vi "Version_2.0_Single_Column_Code.vi"() -> ()   [LabVIEW 2020] (continued)
                              frame #2 {
                                n5157 = local read "VISA Refnum in\nfor Pump"() -> (w5540:refnum<visa-resource-name>)
                                n5158 = call "PortChanger (SubVI).vi"("Port Number"="1", "VISA Refnum in"=w5540) -> ()  [unwired: 10 in]
                              }
                              frame #3 {
                                n5159 = local read "Stopper that ends \nthe main loops"() -> (w5541:bool)
                                n5160 = local read "VISA Refnum in\nfor Pump"() -> (w5542:refnum<visa-resource-name>)
                                n5161 = case shown="True" w5541 {
                                frame False {
                                }
                                frame True {
                                n5162 = local read "VISA Refnum in\nfor Pump"() -> (w5543:refnum<visa-resource-name>)
                                n5163 = call "HardStopCurrentProcess (SubVI).vi"("VISA Refnum in"=w5543) -> ()  [unwired: 11 in]
                                }
                                }
                                n5164 = call "ProcessCompletionWaiter (SubVI).vi"("VISA Refnum in"=w5542) -> ()  [unwired: 11 in]
                              }
                              frame #4 {
                                n5165 = local read "VISA Refnum in\nfor Pump"() -> (w5548:refnum<visa-resource-name>)
                                n5166 = local read "Volume of Syringe"() -> (w5545:dbl)
                                n5167 = call "GoToAbsolutePosition(SubVI).vi"("Absolute Volume Position in Syringe (in ul)"=0.0, "Volume of Syringe"=w5545, "Resolution of Pumping"=T2."Standard Pumping", "Flow Rate (ul/min)"=150.0, "VISA Refnum in"=w5548) -> ()  [unwired: 6 in, 1 out]
                              }
                              frame #5 {
                                n5168 = local read "Stopper that ends \nthe main loops"() -> (w5549:bool)
                                n5169 = local read "VISA Refnum in\nfor Pump"() -> (w5550:refnum<visa-resource-name>)
                                n5170 = case shown="True" w5549 {
                                frame False {
                                }
                                frame True {
                                n5171 = local read "VISA Refnum in\nfor Pump"() -> (w5551:refnum<visa-resource-name>)
                                n5172 = call "HardStopCurrentProcess (SubVI).vi"("VISA Refnum in"=w5551) -> ()  [unwired: 11 in]
                                }
                                }
                                n5173 = call "ProcessCompletionWaiter (SubVI).vi"("VISA Refnum in"=w5550) -> ()  [unwired: 11 in]
                              }
                            }
                          }
                          frame #3 {
                            n5174 = local read "VISA Refnum in\nfor Pump"() -> (w5553:refnum<visa-resource-name>)
                            n5175 = local read "Port for \nB-Elution"() -> (w5552:string)
                            n5176 = call "PortChanger (SubVI).vi"("Port Number"=w5552, "VISA Refnum in"=w5553) -> ()  [unwired: 10 in]
                          }
                          frame #4 {
                            n5177 = local read "VISA Refnum in\nfor Pump"() -> (w5554:refnum<visa-resource-name>)
                            n5178 = call "ProcessCompletionWaiter (SubVI).vi"("VISA Refnum in"=w5554) -> ()  [unwired: 11 in]
                          }
                          frame #5 {
                            n5179 = local read "Buffer-B PickUp \nFlow Rate (ul/min)"() -> (w5557:dbl)
                            n5180 = local read "Buffer-B Pumping\nResolution"() -> (w5556:T2)
                            n5181 = local read "VISA Refnum in\nfor Pump"() -> (w5559:refnum<visa-resource-name>)
                            n5182 = local read "Buffer-B Volume \nto be  Pumped"() -> (w5555:dbl)
                            n5183 = local read "Volume of Syringe"() -> (w5558:dbl)
                            n5184 = call "RPickUp(SubVI).vi"("Volume to be picked up"=w5555, "Volume of Syringe"=w5558, "Resolution of PickUP"=w5556, "PickUp Flow Rate (ul/min)"=w5557, "VISA Refnum in"=w5559) -> ()  [unwired: 6 in, 1 out]
                          }
                          frame #6 {
                            n5185 = local read "Stopper that ends \nthe main loops"() -> (w5560:bool)
                            n5186 = local read "VISA Refnum in\nfor Pump"() -> (w5561:refnum<visa-resource-name>)
                            n5187 = case shown="True" w5560 {
                              frame False {
                              }
                              frame True {
                                n5188 = local read "VISA Refnum in\nfor Pump"() -> (w5562:refnum<visa-resource-name>)
                                n5189 = call "HardStopCurrentProcess (SubVI).vi"("VISA Refnum in"=w5562) -> ()  [unwired: 11 in]
                              }
                            }
                            n5190 = call "ProcessCompletionWaiter (SubVI).vi"("VISA Refnum in"=w5561) -> ()  [unwired: 11 in]
                          }
                          frame #7 {
                            # "Reads the initial Plunger Position for computing the volume dispensed"
                            n5191 = local read "VISA Refnum in\nfor Pump"() -> (w5564:refnum<visa-resource-name>)
                            n5192 = call "AbsolutePlungerPosition (SubVI).vi"("VISA Refnum in"=w5564) -> ("Plunger Position"=w5563:i32)  [unwired: 10 in]
                            n5193 = local write "Initial Plunger Position"(w5563) -> ()
                          }
                          frame #8 {
                            # "Switch to Port-8"
                            # "Port-8 of the pump is conncted to elution port of column-1 of chip"
                            n5194 = local read "VISA Refnum in\nfor Pump"() -> (w5566:refnum<visa-resource-name>)
                            n5195 = call "PortChanger (SubVI).vi"("Port Number"="8", "VISA Refnum in"=w5566) -> ()  [unwired: 10 in]
                          }
                          frame #9 {
                            n5196 = local read "Stopper that ends \nthe main loops"() -> (w5567:bool)
                            n5197 = local read "VISA Refnum in\nfor Pump"() -> (w5568:refnum<visa-resource-name>)
                            n5198 = call "ProcessCompletionWaiter (SubVI).vi"("VISA Refnum in"=w5568) -> ()  [unwired: 11 in]
                            n5199 = case shown="True" w5567 {
                              frame False {
                              }
                              frame True {
                                n5200 = local read "VISA Refnum in\nfor Pump"() -> (w5569:refnum<visa-resource-name>)
                                n5201 = call "HardStopCurrentProcess (SubVI).vi"("VISA Refnum in"=w5569) -> ()  [unwired: 11 in]
                              }
                            }
                          }
                          frame #10 {
                            # "Discard first few microlitres of elution buffer"
                            # "Keeps the AMF valve after column-1 open and valve after column-2 closed"
                            n5202 = local write "Valve V1 Open"(FALSE ("Valve V1 Open")) -> ()
                            n5203 = local write "Valve V2 Open"(FALSE ("Valve V2 Open")) -> ()
                            n5204 = local write "Valve V3 Open"(FALSE ("Valve V3 Open")) -> ()
                            n5205 = local write "Valve V4 Open"(FALSE ("Valve V4 Open")) -> ()
                            n5206 = local write "External Valve \nOpen"(FALSE ("External Valve \nOpen")) -> ()
                            n5207 = local write "Valve V8 Open"(TRUE ("Valve V8 Open")) -> ()
                            n5208 = local write "Valve V6 Open"(FALSE ("Valve V6 Open")) -> ()
                            n5209 = local write "Valve V5 Open"(FALSE ("Valve V5 Open")) -> ()
                            n5210 = local write "Valve V7 Open"(FALSE ("Valve V7 Open")) -> ()
                          }
                          frame #11 {
                            n5211 = local read "Buffer-B Dispense\nFlow Rate (ul/min)"() -> (w5584:dbl)
                            n5212 = local read "Buffer-B Pumping\nResolution"() -> (w5583:T2)
                            n5213 = local read "Initial Plunger Position"() -> (w5580:dbl)
                            n5214 = local read "VISA Refnum in\nfor Pump"() -> (w5586:refnum<visa-resource-name>)
                            n5215 = local read "Volume of Syringe"() -> (w5585:dbl)
                            n5216 = call "GoToAbsolutePosition(SubVI).vi"("Absolute Volume Position in Syringe (in ul)"=0.0 ("Volume to be Dispensed"), "Volume of Syringe"=w5585, "Resolution of Pumping"=w5583, "Flow Rate (ul/min)"=w5584, "VISA Refnum in"=w5586) -> ()  [unwired: 6 in, 1 out]
                            n5217 = local write "Pause Data Collection"(FALSE ("Pause Data Collection")) -> ()
                            n5218 = local write "Vol_now"(0.0 ("Vol_now")) -> ()
                            n5219 = local write "Position\nNow"(w5580) -> ()
                          }
                          frame #12 {
                            n5220 = local read "Buffer-B Pumping\nResolution"() -> (w5591:T2)
                            n5221 = local read "VISA Refnum in\nfor Pump"() -> (w5592:refnum<visa-resource-name>)
                            n5222 = local read "Volume of Syringe"() -> (w5590:dbl)
                            n5223 = local read "Position\nNow"() -> (w5587:dbl)
                            n5224 = local read "Pause Elution"() -> (w5588:bool)
                            n5225 = case shown="False" w5588 {
                              tunnel: w5587 -> [w5596 _]
                              tunnel: w5592 -> [w5595 w5637]
                              tunnel: w5591 -> [w5594 _]
                              tunnel: w5590 -> [w5593 _]
                              frame False {
                                n5226 = stacked-sequence {
                                tunnel: w5596 -> [_ w5602]
                                tunnel: w5595 -> [_ w5601]
                                tunnel: w5594 -> [_ w5600]
                                tunnel: w5593 -> [_ w5599]
                                frame #0 {
                                n5227 = Wait (ms)(milliseconds to wait=u32 3000) -> ()  [unwired: 1 out]
                                n5228 = local write "Signal"(TRUE ("Signal")) -> ()
                                }
                                frame #1 {
                                n5229 = while {
                                tunnel: w5602 -> [w5613]
                                tunnel: w5601 -> [w5612]
                                tunnel: w5600 -> [w5611]
                                tunnel: w5599 -> [w5610]
                                stop <- w5606 stop-if-true
                                n5230 = stacked-sequence {
                                tunnel: w5613 -> [_ w5620]
                                tunnel: w5612 -> [_ w5619]
                                tunnel: w5611 -> [_ w5618]
                                tunnel: w5610 -> [_ w5617]
                                frame #0 {
                                n5231 = Wait (ms)(milliseconds to wait=u32 500) -> ()  [unwired: 1 out]
                                }
                                frame #1 {
                                n5232 = call "AbsolutePlungerPosition (SubVI).vi"("VISA Refnum in"=w5619) -> ("Plunger Position"=w5616:i32)  [unwired: 10 in]
                                n5233 = case shown="\"High Resolution Pumping\"" w5618 {
                                tunnel: w5620 -> [w5625 w5634]
                                tunnel: w5616 -> [w5626 w5633]
                                tunnel: [w5624 w5631] -> w5615
                                tunnel: w5617 -> [w5623 w5632]
                                frame "Standard Pumping", Default {
                                n5234 = Subtract(x=w5625, y=w5626) -> (x-y=w5622:dbl)
                                n5235 = Absolute Value(x=w5622) -> (abs(x)=w5621:dbl)
                                n5236 = Multiply(x=w5621, y=w5623) -> (x*y=w5628:dbl)
                                n5237 = Divide(x=w5628, y=3000.0) -> (x/y=w5624:dbl)
                                }
                                frame "High Resolution Pumping" {
                                n5238 = Subtract(x=w5634, y=w5633) -> (x-y=w5630:dbl)
                                n5239 = Absolute Value(x=w5630) -> (abs(x)=w5629:dbl)
                                n5240 = Multiply(x=w5629, y=w5632) -> (x*y=w5636:dbl)
                                n5241 = Divide(x=w5636, y=24000.0) -> (x/y=w5631:dbl)
                                }
                                }
                                n5242 = local write "Volume being Injected \nin this process"(w5615) -> ()
                                }
                                }
                                n5243 = local read "Volume being Injected \nin this process"() -> (w5604:dbl)
                                n5244 = local read "Discard volume \npriot to elution"() -> (w5605:dbl)
                                n5245 = local read "Divert Elution Buffer\ninto Column-1"() -> (w5609:bool)
                                n5246 = local read "Stopper that ends \nthe main loops"() -> (w5608:bool)
                                n5247 = Greater Or Equal?(x=w5604, y=w5605) -> (x >= y?=w5603:bool)
                                n5248 = Or(x=w5609, y=w5608) -> (x .or. y?=w5607:bool)
                                n5249 = Or(x=w5603, y=w5607) -> (x .or. y?=w5606:bool)
                                }
                                }
                                }
                              }
                              frame True {
                                n5250 = stacked-sequence {
                                tunnel: w5637 -> [_ w5640 _]
                                frame #0 {
                                n5251 = Wait (ms)(milliseconds to wait=u32 2000) -> ()  [unwired: 1 out]
                                }
                                frame #1 {
                                n5252 = local read "Signal"() -> (w5639:bool)
                                n5253 = case shown="True" w5639 {
                                tunnel: w5640 -> [_ w5646]
                                frame False {
                                }
                                frame True {
                                n5254 = local read "Volume being Injected \nin this process"() -> (w5644:dbl)
                                n5255 = local read "Net Elution \nVolume"() -> (w5643:dbl)
                                n5256 = local write "Signal"(FALSE ("Signal")) -> ()
                                n5257 = Add(x=w5644, y=w5643) -> (x+y=w5642:dbl)
                                n5258 = call "AbsolutePlungerPosition (SubVI).vi"("VISA Refnum in"=w5646) -> ("Plunger Position"=w5645:i32)  [unwired: 10 in]
                                n5259 = local write "Net Elution \nVolume"(w5642) -> ()
                                n5260 = local write "Position\nNow"(w5645) -> ()
                                }
                                }
                                }
                                frame #2 {
                                n5261 = local write "Volume being Injected \nin this process"(0.0 ("Volume being Injected \nin this process")) -> ()
                                }
                                }
                              }
                            }
                            n5262 = local read "Stopper that ends \nthe main loops"() -> (w5589:bool)
                            n5263 = case shown="True" w5589 {
                              frame False {
                              }
                              frame True {
                                n5264 = local read "VISA Refnum in\nfor Pump"() -> (w5648:refnum<visa-resource-name>)
                                n5265 = call "HardStopCurrentProcess (SubVI).vi"("VISA Refnum in"=w5648) -> ()  [unwired: 11 in]
                              }
                            }
                          }
                          frame #13 {
                            # "Keeps the AMF valve after column-1 open and valve after column-2 closed"
                            n5266 = local write "Valve V1 Open"(TRUE ("Valve V1 Open")) -> ()
                            n5267 = local write "Valve V2 Open"(TRUE ("Valve V2 Open")) -> ()
                            n5268 = local write "Valve V3 Open"(FALSE ("Valve V3 Open")) -> ()
                            n5269 = local write "Valve V4 Open"(FALSE ("Valve V4 Open")) -> ()
                            n5270 = local write "External Valve \nOpen"(TRUE ("External Valve \nOpen")) -> ()
                            n5271 = local write "Valve V8 Open"(FALSE ("Valve V8 Open")) -> ()
                            n5272 = local write "Valve V6 Open"(FALSE ("Valve V6 Open")) -> ()
                            n5273 = local write "Valve V5 Open"(FALSE ("Valve V5 Open")) -> ()
                            n5274 = local write "Valve V7 Open"(FALSE ("Valve V7 Open")) -> ()
                          }
                          frame #14 {
                            n5275 = while {
                              stop <- w5664 stop-if-true
                              n5276 = event shown="[1] \"Divert Sample  into Column-2\": Value Change" {
                                selector: _ -> [_ _ _ _]
                                dyn-events: _ -> [_ _ _ _]
                                timeout: 100 -> [_ _ _ _]
                                tunnel: [_ _ w5679 _] -> w5663
                                tunnel: [_ w5678 _ _] -> w5662
                                event "Pause Elution\nValue": Value Change {
                                n5277 = event-data() -> ()  [unwired: 1 in, 6 out]
                                n5278 = stacked-sequence {
                                frame #0 {
                                n5279 = local read "Pause Elution"() -> (w5666:bool)
                                n5280 = case shown="False" w5666 {
                                frame False {
                                n5281 = local write "Pause Elution"(TRUE ("Pause Elution")) -> ()
                                }
                                frame True {
                                n5282 = local write "Pause Elution"(FALSE ("Pause Elution")) -> ()
                                }
                                }
                                }
                                frame #1 {
                                n5283 = local read "Pause Elution"() -> (w5669:bool)
                                n5284 = case shown="False" w5669 {
                                frame False {
                                n5285 = local read "Buffer-B Dispense\nFlow Rate (ul/min)"() -> (w5674:dbl)
                                n5286 = local read "VISA Refnum in\nfor Pump"() -> (w5675:refnum<visa-resource-name>)
                                n5287 = local read "Buffer-B Pumping\nResolution"() -> (w5671:T2)
                                n5288 = local read "Volume of Syringe"() -> (w5672:dbl)
                                n5289 = call "GoToAbsolutePosition(SubVI).vi"("Absolute Volume Position in Syringe (in ul)"=0.0, "Volume of Syringe"=w5672, "Resolution of Pumping"=w5671, "Flow Rate (ul/min)"=w5674, "VISA Refnum in"=w5675) -> ()  [unwired: 6 in, 1 out]
                                n5290 = local write "Pause Data Collection"(FALSE ("Pause Data Collection")) -> ()
                                }
                                frame True {
                                n5291 = local read "VISA Refnum in\nfor Pump"() -> (w5677:refnum<visa-resource-name>)
                                n5292 = local write "Pause Data Collection"(TRUE ("Pause Data Collection")) -> ()
                                n5293 = call "HardStopCurrentProcess (SubVI).vi"("VISA Refnum in"=w5677) -> ()  [unwired: 11 in]
                                }
                                }
                                }
                                }
                                }
                                event "Divert Sample \ninto Column-2": Value Change {
                                n5294 = event-data() -> ()  [unwired: 1 in, 6 out]
                                n5295 = local read "Divert Sample \ninto Column-2"() -> (w5678:bool)
                                }
                                event "Stop for End of \nExperiment \nand Data Writing": Value Change {
                                n5296 = event-data() -> ()  [unwired: 1 in, 6 out]
                                n5297 = local read "Stop for End of \nExperiment \nand Data Writing"() -> (w5679:bool)
                                }
                                event Timeout {
                                n5298 = event-data() -> ()  [unwired: 1 in, 3 out]
                                }
                              }
                              n5299 = Or(x=w5662, y=w5663) -> (x .or. y?=w5664:bool)
                            }
                            n5300 = local read "Buffer-B Pumping\nResolution"() -> (w5660:T2)
                            n5301 = local read "VISA Refnum in\nfor Pump"() -> (w5661:refnum<visa-resource-name>)
                            n5302 = local read "Volume of Syringe"() -> (w5659:dbl)
                            n5303 = while {
                              tunnel: w5661 -> [w5688]
                              tunnel: w5660 -> [w5687]
                              tunnel: w5659 -> [w5686]
                              stop <- w5682 stop-if-true
                              n5304 = local read "Position\nNow"() -> (w5680:dbl)
                              n5305 = local read "Pause Elution"() -> (w5681:bool)
                              n5306 = case shown="False" w5681 {
                                tunnel: w5680 -> [w5692 _]
                                tunnel: w5688 -> [w5691 w5734]
                                tunnel: w5687 -> [w5690 _]
                                tunnel: w5686 -> [w5689 _]
                                frame False {
                                n5307 = stacked-sequence {
                                tunnel: w5692 -> [_ w5698]
                                tunnel: w5691 -> [_ w5697]
                                tunnel: w5690 -> [_ w5696]
                                tunnel: w5689 -> [_ w5695]
                                frame #0 {
                                n5308 = Wait (ms)(milliseconds to wait=u32 3000) -> ()  [unwired: 1 out]
                                n5309 = local write "Signal"(TRUE ("Signal")) -> ()
                                }
                                frame #1 {
                                n5310 = while {
                                tunnel: w5698 -> [w5710]
                                tunnel: w5697 -> [w5709]
                                tunnel: w5696 -> [w5708]
                                tunnel: w5695 -> [w5707]
                                stop <- w5702 stop-if-true
                                n5311 = stacked-sequence {
                                tunnel: w5710 -> [_ w5717]
                                tunnel: w5709 -> [_ w5716]
                                tunnel: w5708 -> [_ w5715]
                                tunnel: w5707 -> [_ w5714]
                                frame #0 {
                                n5312 = Wait (ms)(milliseconds to wait=u32 500) -> ()  [unwired: 1 out]
                                }
                                frame #1 {
                                n5313 = call "AbsolutePlungerPosition (SubVI).vi"("VISA Refnum in"=w5716) -> ("Plunger Position"=w5713:i32)  [unwired: 10 in]
                                n5314 = case shown="\"High Resolution Pumping\"" w5715 {
                                tunnel: w5717 -> [w5722 w5731]
                                tunnel: w5713 -> [w5723 w5730]
                                tunnel: [w5721 w5728] -> w5712
                                tunnel: w5714 -> [w5720 w5729]
                                frame "Standard Pumping", Default {
                                n5315 = Subtract(x=w5722, y=w5723) -> (x-y=w5719:dbl)
                                n5316 = Absolute Value(x=w5719) -> (abs(x)=w5718:dbl)
                                n5317 = Multiply(x=w5718, y=w5720) -> (x*y=w5725:dbl)
                                n5318 = Divide(x=w5725, y=3000.0) -> (x/y=w5721:dbl)
                                }
                                frame "High Resolution Pumping" {
                                n5319 = Subtract(x=w5731, y=w5730) -> (x-y=w5727:dbl)
                                n5320 = Absolute Value(x=w5727) -> (abs(x)=w5726:dbl)
                                n5321 = Multiply(x=w5726, y=w5729) -> (x*y=w5733:dbl)
                                n5322 = Divide(x=w5733, y=24000.0) -> (x/y=w5728:dbl)
                                }
                                }
                                n5323 = local write "Volume being Injected \nin this process"(w5712) -> ()
                                }
                                }
                                n5324 = local read "Volume being Injected \nin this process"() -> (w5700:dbl)
                                n5325 = local read "Affinity Elution \nGraph Min CutOff"() -> (w5699:dbl)
                                n5326 = local read "Stopper that ends \nthe main loops"() -> (w5705:bool)
                                n5327 = local read "Divert Sample \ninto Column-2"() -> (w5706:bool)
                                n5328 = Greater Or Equal?(x=w5700, y=w5699) -> (x >= y?=w5701:bool)
                                n5329 = Or(x=w5706, y=w5705) -> (x .or. y?=w5703:bool)
                                n5330 = local read "Pause Elution"() -> (w5704:bool)
                                n5331 = local write "Affinity Elution \nis Approaching"(w5701) -> ()
                                n5332 = Or(x=w5704, y=w5703) -> (x .or. y?=w5702:bool)
                                }
                                }
                                }
                                }
                                frame True {
                                n5333 = stacked-sequence {
                                tunnel: w5734 -> [_ w5737 _]
                                frame #0 {
                                n5334 = Wait (ms)(milliseconds to wait=u32 2000) -> ()  [unwired: 1 out]
                                }
                                frame #1 {
                                n5335 = local read "Signal"() -> (w5736:bool)
                                n5336 = case shown="True" w5736 {
                                tunnel: w5737 -> [_ w5743]
                                frame False {
                                }
                                frame True {
                                n5337 = local read "Volume being Injected \nin this process"() -> (w5741:dbl)
                                n5338 = local read "Net Elution \nVolume"() -> (w5740:dbl)
                                n5339 = local write "Signal"(FALSE ("Signal")) -> ()
                                n5340 = Add(x=w5741, y=w5740) -> (x+y=w5739:dbl)
                                n5341 = call "AbsolutePlungerPosition (SubVI).vi"("VISA Refnum in"=w5743) -> ("Plunger Position"=w5742:i32)  [unwired: 10 in]
                                n5342 = local write "Net Elution \nVolume"(w5739) -> ()
                                n5343 = local write "Position\nNow"(w5742) -> ()
                                }
                                }
                                }
                                frame #2 {
                                n5344 = local write "Volume being Injected \nin this process"(0.0 ("Volume being Injected \nin this process")) -> ()
                                }
                                }
                                }
                              }
                              n5345 = local read "Stopper that ends \nthe main loops"() -> (w5684:bool)
                              n5346 = local read "Divert Sample \ninto Column-2"() -> (w5683:bool)
                              n5347 = Or(x=w5683, y=w5684) -> (x .or. y?=w5682:bool)
                              n5348 = Wait (ms)(milliseconds to wait=u32 300) -> ()  [unwired: 1 out]
                            }
                            n5349 = local read "Stopper that ends \nthe main loops"() -> (w5658:bool)
                            n5350 = case shown="True" w5658 {
                              frame False {
                              }
                              frame True {
                                n5351 = local read "VISA Refnum in\nfor Pump"() -> (w5745:refnum<visa-resource-name>)
                                n5352 = call "HardStopCurrentProcess (SubVI).vi"("VISA Refnum in"=w5745) -> ()  [unwired: 11 in]
                              }
                            }
                          }
                          frame #15 {
                            # "Keeps the on-chip Valve V1 and V3 after column-2 open"
                            # "Keeps the AMF valve after column-1 closed and valve after column-2 open"
                            n5353 = local read "VISA Refnum in\nfor Pump"() -> (w5758:refnum<visa-resource-name>)
                            n5354 = local read "Volume being Injected \nin this process"() -> (w5755:dbl)
                            n5355 = local write "Sample Volume Diverted\ninto Column-2"(0.0 ("Sample Volume Diverted\ninto Column-2")) -> ()
                            n5356 = call "AbsolutePlungerPosition (SubVI).vi"("VISA Refnum in"=w5758) -> ("Plunger Position"=w5757:i32)  [unwired: 10 in]
                            n5357 = local write "Position\nNow"(w5757) -> ()
                            n5358 = local write "Vol_previous"(0.0 ("Vol_diff")) -> ()
                            n5359 = local write "Vol_now"(w5755) -> ()
                            n5360 = local write "Valve V1 Open"(TRUE ("Valve V1 Open")) -> ()
                            n5361 = local write "Valve V3 Open"(FALSE ("Valve V3 Open")) -> ()
                            n5362 = local write "Valve V2 Open"(FALSE ("Valve V2 Open")) -> ()
                            n5363 = local write "Valve V4 Open"(TRUE ("Valve V4 Open")) -> ()
                            n5364 = local write "External Valve \nOpen"(FALSE ("External Valve \nOpen")) -> ()
                            n5365 = local write "Valve V8 Open"(FALSE ("Valve V8 Open")) -> ()
                            n5366 = local write "Valve V5 Open"(TRUE ("Valve V5 Open")) -> ()
                            n5367 = local write "Valve V6 Open"(FALSE ("Valve V6 Open")) -> ()
                            n5368 = local write "Valve V7 Open"(TRUE ("Valve V7 Open")) -> ()
                          }
                          frame #16 {
                            n5369 = local read "Divert Sample \ninto Column-2"() -> (w5760:bool)
                            n5370 = case shown="True" w5760 {
                              frame False {
                                n5371 = stacked-sequence {
                                frame #0 {
                                n5372 = local read "Buffer-B Pumping\nResolution"() -> (w5763:T2)
                                n5373 = local read "VISA Refnum in\nfor Pump"() -> (w5765:refnum<visa-resource-name>)
                                n5374 = local read "Initial Plunger Position"() -> (w5764:dbl)
                                n5375 = local read "Volume of Syringe"() -> (w5762:dbl)
                                n5376 = while {
                                tunnel: w5764 -> [w5771]
                                tunnel: w5765 -> [w5770]
                                tunnel: w5763 -> [w5769]
                                tunnel: w5762 -> [w5768]
                                stop <- w5766 stop-if-true
                                n5377 = Wait (ms)(milliseconds to wait=u32 100) -> ()  [unwired: 1 out]
                                n5378 = stacked-sequence {
                                tunnel: w5771 -> [w5777 _]
                                tunnel: w5770 -> [w5776 w5797]
                                tunnel: w5769 -> [w5775 _]
                                tunnel: w5768 -> [w5774 _]
                                tunnel: [_ w5795] -> w5766
                                frame #0 {
                                n5379 = call "AbsolutePlungerPosition (SubVI).vi"("VISA Refnum in"=w5776) -> ("Plunger Position"=w5773:i32)  [unwired: 10 in]
                                n5380 = case shown="\"Standard Pumping\", Default" w5775 {
                                tunnel: w5777 -> [w5782 w5791]
                                tunnel: w5773 -> [w5783 w5790]
                                tunnel: [w5781 w5788] -> w5772
                                tunnel: w5774 -> [w5780 w5789]
                                frame "Standard Pumping", Default {
                                n5381 = Subtract(x=w5782, y=w5783) -> (x-y=w5779:dbl)
                                n5382 = Absolute Value(x=w5779) -> (abs(x)=w5778:dbl)
                                n5383 = Multiply(x=w5778, y=w5780) -> (x*y=w5785:dbl)
                                n5384 = Divide(x=w5785, y=3000.0) -> (x/y=w5781:dbl)
                                }
                                frame "High Resolution Pumping" {
                                n5385 = Subtract(x=w5791, y=w5790) -> (x-y=w5787:dbl)
                                n5386 = Absolute Value(x=w5787) -> (abs(x)=w5786:dbl)
                                n5387 = Multiply(x=w5786, y=w5789) -> (x*y=w5793:dbl)
                                n5388 = Divide(x=w5793, y=24000.0) -> (x/y=w5788:dbl)
                                }
                                }
                                n5389 = local write "Volume being Injected \nin this process"(w5772) -> ()
                                }
                                frame #1 {
                                n5390 = local read "Stopper that ends \nthe main loops"() -> (w5794:bool)
                                n5391 = call "LSPOneStatus (SubVI).vi"("VISA Refnum in"=w5797) -> ("read buffer"=w5799:string)  [unwired: 10 in]
                                n5392 = call <vilib>:"Trim Whitespace.vi"("string"=w5799) -> ("trimmed string"=w5798:string)  [unwired: 1 in]
                                n5393 = Equal?(x=w5798, y="/0`\u0003") -> (x = y?=w5796:bool)
                                n5394 = Or(x=w5796, y=w5794) -> (x .or. y?=w5795:bool)
                                }
                                }
                                }
                                n5395 = local read "Stopper that ends \nthe main loops"() -> (w5761:bool)
                                n5396 = case shown="True" w5761 {
                                frame False {
                                }
                                frame True {
                                n5397 = local read "VISA Refnum in\nfor Pump"() -> (w5801:refnum<visa-resource-name>)
                                n5398 = call "HardStopCurrentProcess (SubVI).vi"("VISA Refnum in"=w5801) -> ()  [unwired: 11 in]
                                }
                                }
                                }
                                }
                              }
                              frame True {
                                n5399 = stacked-sequence {
                                frame #0 {
                                n5400 = local read "Buffer-B Pumping\nResolution"() -> (w5804:T2)
                                n5401 = local read "VISA Refnum in\nfor Pump"() -> (w5806:refnum<visa-resource-name>)
                                n5402 = local read "Volume of Syringe"() -> (w5803:dbl)
                                n5403 = local read "Position\nNow"() -> (w5805:dbl)
                                n5404 = while {
                                tunnel: w5805 -> [w5812]
                                tunnel: w5806 -> [w5811]
                                tunnel: w5804 -> [w5810]
                                tunnel: w5803 -> [w5809]
                                stop <- w5807 stop-if-true
                                n5405 = Wait (ms)(milliseconds to wait=u32 100) -> ()  [unwired: 1 out]
                                n5406 = stacked-sequence {
                                tunnel: w5812 -> [w5822 _ _]
                                tunnel: w5811 -> [w5821 _ w5848]
                                tunnel: w5810 -> [w5820 _ _]
                                tunnel: w5809 -> [w5819 _ _]
                                tunnel: [_ _ w5846] -> w5807
                                frame #0 {
                                n5407 = local read "Vol_previous"() -> (w5816:dbl)
                                n5408 = call "AbsolutePlungerPosition (SubVI).vi"("VISA Refnum in"=w5821) -> ("Plunger Position"=w5818:i32)  [unwired: 10 in]
                                n5409 = case shown="\"Standard Pumping\", Default" w5820 {
                                tunnel: w5822 -> [w5827 w5836]
                                tunnel: w5818 -> [w5828 w5835]
                                tunnel: [w5826 w5833] -> w5817
                                tunnel: w5819 -> [w5825 w5834]
                                frame "Standard Pumping", Default {
                                n5410 = Subtract(x=w5827, y=w5828) -> (x-y=w5824:dbl)
                                n5411 = Absolute Value(x=w5824) -> (abs(x)=w5823:dbl)
                                n5412 = Multiply(x=w5823, y=w5825) -> (x*y=w5830:dbl)
                                n5413 = Divide(x=w5830, y=3000.0) -> (x/y=w5826:dbl)
                                }
                                frame "High Resolution Pumping" {
                                n5414 = Subtract(x=w5836, y=w5835) -> (x-y=w5832:dbl)
                                n5415 = Absolute Value(x=w5832) -> (abs(x)=w5831:dbl)
                                n5416 = Multiply(x=w5831, y=w5834) -> (x*y=w5838:dbl)
                                n5417 = Divide(x=w5838, y=24000.0) -> (x/y=w5833:dbl)
                                }
                                }
                                n5418 = Subtract(x=w5817, y=w5816) -> (x-y=w5815:dbl)
                                n5419 = local read "Vol_now"() -> (w5813:dbl)
                                n5420 = local write "Sample Volume Diverted\ninto Column-2"(w5817) -> ()
                                n5421 = Add(x=w5815, y=w5813) -> (x+y=w5814:dbl)
                                n5422 = local write "Volume being Injected \nin this process"(w5814) -> ()
                                }
                                frame #1 {
                                n5423 = local read "Volume being Injected \nin this process"() -> (w5839:dbl)
                                n5424 = local read "Sample Volume Diverted\ninto Column-2"() -> (w5840:dbl)
                                n5425 = local write "Vol_now"(w5839) -> ()
                                n5426 = local write "Vol_previous"(w5840) -> ()
                                }
                                frame #2 {
                                n5427 = local read "Buffer-B Volume \nto be Pumped for\nSample Diversion\nto Column-2"() -> (w5842:dbl)
                                n5428 = local read "Sample Volume Diverted\ninto Column-2"() -> (w5841:dbl)
                                n5429 = local read "Stopper that ends \nthe main loops"() -> (w5843:bool)
                                n5430 = call "LSPOneStatus (SubVI).vi"("VISA Refnum in"=w5848) -> ("read buffer"=w5850:string)  [unwired: 10 in]
                                n5431 = call <vilib>:"Trim Whitespace.vi"("string"=w5850) -> ("trimmed string"=w5849:string)  [unwired: 1 in]
                                n5432 = Equal?(x=w5849, y="/0`\u0003") -> (x = y?=w5847:bool)
                                n5433 = Greater Or Equal?(x=w5841, y=w5842) -> (x >= y?=w5845:bool)
                                n5434 = Or(x=w5843, y=w5845) -> (x .or. y?=w5844:bool)
                                n5435 = Or(x=w5847, y=w5844) -> (x .or. y?=w5846:bool)
                                }
                                }
                                }
                                n5436 = local read "Stopper that ends \nthe main loops"() -> (w5802:bool)
                                n5437 = case shown="True" w5802 {
                                frame False {
                                }
                                frame True {
                                n5438 = local read "VISA Refnum in\nfor Pump"() -> (w5852:refnum<visa-resource-name>)
                                n5439 = call "HardStopCurrentProcess (SubVI).vi"("VISA Refnum in"=w5852) -> ()  [unwired: 11 in]
                                }
                                }
                                }
                                frame #1 {
                                n5440 = local read "VISA Refnum in\nfor Pump"() -> (w5854:refnum<visa-resource-name>)
                                n5441 = local write "Pause Data Collection"(TRUE ("Pause Data Collection")) -> ()
                                n5442 = call "HardStopCurrentProcess (SubVI).vi"("VISA Refnum in"=w5854) -> ()  [unwired: 11 in]
                                }
                                frame #2 {
                                n5443 = local read "VISA Refnum in\nfor Pump"() -> (w5855:refnum<visa-resource-name>)
                                n5444 = call "PortChanger (SubVI).vi"("Port Number"="1", "VISA Refnum in"=w5855) -> ()  [unwired: 10 in]
                                }
                                frame #3 {
                                n5445 = local read "VISA Refnum in\nfor Pump"() -> (w5861:refnum<visa-resource-name>)
                                n5446 = local read "Volume of Syringe"() -> (w5857:dbl)
                                n5447 = call "GoToAbsolutePosition(SubVI).vi"("Absolute Volume Position in Syringe (in ul)"=0.0, "Volume of Syringe"=w5857, "Resolution of Pumping"=T2."Standard Pumping", "Flow Rate (ul/min)"=150.0, "VISA Refnum in"=w5861) -> ()  [unwired: 6 in, 1 out]
                                }
                                frame #4 {
                                n5448 = local read "VISA Refnum in\nfor Pump"() -> (w5863:refnum<visa-resource-name>)
                                n5449 = local write "Divert Sample \ninto Column-2"(FALSE ("Divert Sample \ninto Column-2")) -> ()
                                n5450 = call "ProcessCompletionWaiter (SubVI).vi"("VISA Refnum in"=w5863) -> ()  [unwired: 11 in]
                                }
                                }
                              }
                            }
                          }
                          frame #17 {
                            # "Keeps the On-Chip Valves V1 and V3 closed"
                            # "Switch to Port-5/8"
                            # "Port-5/8 of pump is connected to Buffer-C1/C2"
                            # "Keeps the AMF valve after column-1 open and valve after column-2 closed"
                            n5451 = local read "VISA Refnum in\nfor Pump"() -> (w5876:refnum<visa-resource-name>)
                            n5452 = local write "Pause Data Collection"(TRUE ("Pause Data Collection")) -> ()
                            n5453 = Wait (ms)(milliseconds to wait=u32 500) -> ()  [unwired: 1 out]
                            n5454 = local write "Affinity On"(FALSE ("Affinity On")) -> ()
                            n5455 = local read "Port for \nC2-Elution"() -> (w5869:string)
                            n5456 = local write "Affinity Elution On"(FALSE ("Affinity Elution On")) -> ()
                            n5457 = call "PortChanger (SubVI).vi"("Port Number"=w5869, "VISA Refnum in"=w5876) -> ()  [unwired: 10 in]
                            n5458 = local write "Valve V1 Open"(FALSE ("Valve V1 Open")) -> ()
                            n5459 = local write "Valve V2 Open"(FALSE ("Valve V2 Open")) -> ()
                            n5460 = local write "Valve V3 Open"(FALSE ("Valve V3 Open")) -> ()
                            n5461 = local write "Valve V4 Open"(FALSE ("Valve V4 Open")) -> ()
                            n5462 = local write "External Valve \nOpen"(FALSE ("External Valve \nOpen")) -> ()
                            n5463 = local write "Valve V8 Open"(FALSE ("Valve V8 Open")) -> ()
                            n5464 = local write "Valve V5 Open"(FALSE ("Valve V5 Open")) -> ()
                            n5465 = local write "Valve V6 Open"(FALSE ("Valve V6 Open")) -> ()
                            n5466 = local write "Valve V7 Open"(FALSE ("Valve V7 Open")) -> ()
                          }
                          frame #18 {
                            n5467 = local read "VISA Refnum in\nfor Pump"() -> (w5880:refnum<visa-resource-name>)
                            n5468 = call "ProcessCompletionWaiter (SubVI).vi"("VISA Refnum in"=w5880) -> ()  [unwired: 11 in]
                            n5469 = local write "Start the Process"(FALSE ("Start the Process")) -> ()
                          }
                          frame #19 {
                            n5470 = local read "Stopper that ends \nthe main loops"() -> (w5884:bool)
                            n5471 = local read "Start the Process"() -> (w5885:bool)
                            n5472 = Or(x=w5885, y=w5884) -> (x .or. y?=w5883:bool)
                            n5473 = local write "Elution of Column-1"(FALSE ("Elution of Column-1")) -> ()
                            n5474 = case shown="False" w5883 {
                              frame False {
                                n5475 = while {
                                stop <- w5889 stop-if-true
                                n5476 = local read "Stopper that ends \nthe main loops"() -> (w5890:bool)
                                n5477 = local read "Start the Process"() -> (w5891:bool)
                                n5478 = Or(x=w5891, y=w5890) -> (x .or. y?=w5889:bool)
                                n5479 = Wait (ms)(milliseconds to wait=u32 10) -> ()  [unwired: 1 out]
                                }
                                n5480 = One Button Dialog(message="Move to Column-2 detection zone and Press 'Start the Process' Button.") -> ()  [unwired: 1 in, 1 out]
                              }
                              frame True {
                              }
                            }
                            n5481 = local write "Volume being Injected \nin this process"(0.0 ("Volume being Injected \nin this process")) -> ()
                            n5482 = local write "Elution of Column-2"(TRUE ("Elution of Column-2")) -> ()
                          }
                          frame #20 {
                            # "If Yes, it will clean the SEC buffer from port-8 tubing else it will clean the pump valve a bit"
                            n5483 = local read "Clean the \nBuffer-C2 tubing"() -> (w5892:bool)
                            n5484 = case shown="False" w5892 {
                              frame False {
                                n5485 = stacked-sequence {
                                frame #0 {
                                n5486 = local read "VISA Refnum in\nfor Pump"() -> (w5894:refnum<visa-resource-name>)
                                n5487 = local read "Port for \nC2-Elution"() -> (w5893:string)
                                n5488 = call "PortChanger (SubVI).vi"("Port Number"=w5893, "VISA Refnum in"=w5894) -> ()  [unwired: 10 in]
                                }
                                frame #1 {
                                n5489 = local read "VISA Refnum in\nfor Pump"() -> (w5895:refnum<visa-resource-name>)
                                n5490 = call "ProcessCompletionWaiter (SubVI).vi"("VISA Refnum in"=w5895) -> ()  [unwired: 11 in]
                                }
                                frame #2 {
                                n5491 = local read "Buffer-C2 Pumping\nResolution"() -> (w5898:T2)
                                n5492 = local read "VISA Refnum in\nfor Pump"() -> (w5900:refnum<visa-resource-name>)
                                n5493 = local read "V-S"() -> (w5896:dbl)
                                n5494 = local read "Volume of Syringe"() -> (w5899:dbl)
                                n5495 = call "RPickUp(SubVI).vi"("Volume to be picked up"=w5896, "Volume of Syringe"=w5899, "Resolution of PickUP"=w5898, "PickUp Flow Rate (ul/min)"=150.0, "VISA Refnum in"=w5900) -> ()  [unwired: 6 in, 1 out]
                                }
                                frame #3 {
                                n5496 = local read "Stopper that ends \nthe main loops"() -> (w5901:bool)
                                n5497 = local read "VISA Refnum in\nfor Pump"() -> (w5902:refnum<visa-resource-name>)
                                n5498 = case shown="True" w5901 {
                                frame False {
                                }
                                frame True {
                                n5499 = local read "VISA Refnum in\nfor Pump"() -> (w5903:refnum<visa-resource-name>)
                                n5500 = call "HardStopCurrentProcess (SubVI).vi"("VISA Refnum in"=w5903) -> ()  [unwired: 11 in]
                                }
                                }
                                n5501 = call "ProcessCompletionWaiter (SubVI).vi"("VISA Refnum in"=w5902) -> ()  [unwired: 11 in]
                                }
                                frame #4 {
                                n5502 = local read "VISA Refnum in\nfor Pump"() -> (w5905:refnum<visa-resource-name>)
                                n5503 = call "PortChanger (SubVI).vi"("Port Number"="1", "VISA Refnum in"=w5905) -> ()  [unwired: 10 in]
                                }
                                frame #5 {
                                n5504 = local read "Stopper that ends \nthe main loops"() -> (w5906:bool)
                                n5505 = local read "VISA Refnum in\nfor Pump"() -> (w5907:refnum<visa-resource-name>)
                                n5506 = case shown="True" w5906 {
                                frame False {
                                }
                                frame True {
                                n5507 = local read "VISA Refnum in\nfor Pump"() -> (w5908:refnum<visa-resource-name>)
                                n5508 = call "HardStopCurrentProcess (SubVI).vi"("VISA Refnum in"=w5908) -> ()  [unwired: 11 in]
                                }
                                }
                                n5509 = call "ProcessCompletionWaiter (SubVI).vi"("VISA Refnum in"=w5907) -> ()  [unwired: 11 in]
                                }
                                frame #6 {
                                n5510 = local read "VISA Refnum in\nfor Pump"() -> (w5913:refnum<visa-resource-name>)
                                n5511 = local read "Volume of Syringe"() -> (w5910:dbl)
                                n5512 = call "GoToAbsolutePosition(SubVI).vi"("Absolute Volume Position in Syringe (in ul)"=0.0, "Volume of Syringe"=w5910, "Resolution of Pumping"=T2."Standard Pumping", "Flow Rate (ul/min)"=150.0, "VISA Refnum in"=w5913) -> ()  [unwired: 6 in, 1 out]
                                }
                                frame #7 {
                                n5513 = local read "Stopper that ends \nthe main loops"() -> (w5914:bool)
                                n5514 = local read "VISA Refnum in\nfor Pump"() -> (w5915:refnum<visa-resource-name>)
                                n5515 = case shown="True" w5914 {
                                frame False {
                                }
                                frame True {
                                n5516 = local read "VISA Refnum in\nfor Pump"() -> (w5916:refnum<visa-resource-name>)
                                n5517 = call "HardStopCurrentProcess (SubVI).vi"("VISA Refnum in"=w5916) -> ()  [unwired: 11 in]
                                }
                                }
                                n5518 = call "ProcessCompletionWaiter (SubVI).vi"("VISA Refnum in"=w5915) -> ()  [unwired: 11 in]
                                }
                                }
                              }
                              frame True {
                                n5519 = for {
                                N: 2 -> [_]
                                n5520 = stacked-sequence {
                                frame #0 {
                                n5521 = local read "VISA Refnum in\nfor Pump"() -> (w5919:refnum<visa-resource-name>)
                                n5522 = local read "Port for \nC2-Elution"() -> (w5918:string)
                                n5523 = call "PortChanger (SubVI).vi"("Port Number"=w5918, "VISA Refnum in"=w5919) -> ()  [unwired: 10 in]
                                }
                                frame #1 {
                                n5524 = local read "VISA Refnum in\nfor Pump"() -> (w5920:refnum<visa-resource-name>)
                                n5525 = call "ProcessCompletionWaiter (SubVI).vi"("VISA Refnum in"=w5920) -> ()  [unwired: 11 in]
                                }
                                frame #2 {
                                n5526 = local read "Buffer-C2 Pumping\nResolution"() -> (w5923:T2)
                                n5527 = local read "VISA Refnum in\nfor Pump"() -> (w5925:refnum<visa-resource-name>)
                                n5528 = local read "Apparent Volume\nof Syringe"() -> (w5921:dbl)
                                n5529 = local read "Volume of Syringe"() -> (w5924:dbl)
                                n5530 = call "RPickUp(SubVI).vi"("Volume to be picked up"=w5921, "Volume of Syringe"=w5924, "Resolution of PickUP"=w5923, "PickUp Flow Rate (ul/min)"=150.0, "VISA Refnum in"=w5925) -> ()  [unwired: 6 in, 1 out]
                                }
                                frame #3 {
                                n5531 = local read "Stopper that ends \nthe main loops"() -> (w5926:bool)
                                n5532 = local read "VISA Refnum in\nfor Pump"() -> (w5927:refnum<visa-resource-name>)
                                n5533 = case shown="True" w5926 {
                                frame False {
                                }
                                frame True {
                                n5534 = local read "VISA Refnum in\nfor Pump"() -> (w5928:refnum<visa-resource-name>)
                                n5535 = call "HardStopCurrentProcess (SubVI).vi"("VISA Refnum in"=w5928) -> ()  [unwired: 11 in]
                                }
                                }
                                n5536 = call "ProcessCompletionWaiter (SubVI).vi"("VISA Refnum in"=w5927) -> ()  [unwired: 11 in]
                                }
                                frame #4 {
                                n5537 = local read "VISA Refnum in\nfor Pump"() -> (w5930:refnum<visa-resource-name>)
                                n5538 = call "PortChanger (SubVI).vi"("Port Number"="1", "VISA Refnum in"=w5930) -> ()  [unwired: 10 in]
                                }
                                frame #5 {
                                n5539 = local read "Stopper that ends \nthe main loops"() -> (w5931:bool)
                                n5540 = local read "VISA Refnum in\nfor Pump"() -> (w5932:refnum<visa-resource-name>)
                                n5541 = case shown="True" w5931 {
                                frame False {
                                }
                                frame True {
                                n5542 = local read "VISA Refnum in\nfor Pump"() -> (w5933:refnum<visa-resource-name>)
                                n5543 = call "HardStopCurrentProcess (SubVI).vi"("VISA Refnum in"=w5933) -> ()  [unwired: 11 in]
                                }
                                }
                                n5544 = call "ProcessCompletionWaiter (SubVI).vi"("VISA Refnum in"=w5932) -> ()  [unwired: 11 in]
                                }
                                frame #6 {
                                n5545 = local read "VISA Refnum in\nfor Pump"() -> (w5938:refnum<visa-resource-name>)
                                n5546 = local read "Volume of Syringe"() -> (w5935:dbl)
                                n5547 = call "GoToAbsolutePosition(SubVI).vi"("Absolute Volume Position in Syringe (in ul)"=0.0, "Volume of Syringe"=w5935, "Resolution of Pumping"=T2."Standard Pumping", "Flow Rate (ul/min)"=150.0, "VISA Refnum in"=w5938) -> ()  [unwired: 6 in, 1 out]
                                }
                                frame #7 {
                                n5548 = local read "Stopper that ends \nthe main loops"() -> (w5939:bool)
                                n5549 = local read "VISA Refnum in\nfor Pump"() -> (w5940:refnum<visa-resource-name>)
                                n5550 = case shown="True" w5939 {
                                frame False {
                                }
                                frame True {
                                n5551 = local read "VISA Refnum in\nfor Pump"() -> (w5941:refnum<visa-resource-name>)
                                n5552 = call "HardStopCurrentProcess (SubVI).vi"("VISA Refnum in"=w5941) -> ()  [unwired: 11 in]
                                }
                                }
                                n5553 = call "ProcessCompletionWaiter (SubVI).vi"("VISA Refnum in"=w5940) -> ()  [unwired: 11 in]
                                }
                                }
                                }
                              }
                            }
                          }
                          frame #21 {
                            n5554 = local read "VISA Refnum in\nfor Pump"() -> (w5943:refnum<visa-resource-name>)
                            n5555 = local read "Port for \nC2-Elution"() -> (w5942:string)
                            n5556 = call "PortChanger (SubVI).vi"("Port Number"=w5942, "VISA Refnum in"=w5943) -> ()  [unwired: 10 in]
                          }
                          frame #22 {
                            n5557 = local read "VISA Refnum in\nfor Pump"() -> (w5944:refnum<visa-resource-name>)
                            n5558 = call "ProcessCompletionWaiter (SubVI).vi"("VISA Refnum in"=w5944) -> ()  [unwired: 11 in]
                          }
                          frame #23 {
                            n5559 = local read "Buffer-C2 PickUp \nFlow Rate (ul/min)"() -> (w5948:dbl)
                            n5560 = local read "Buffer-C2 Pumping\nResolution"() -> (w5947:T2)
                            n5561 = local read "VISA Refnum in\nfor Pump"() -> (w5950:refnum<visa-resource-name>)
                            n5562 = local read "Buffer-C2 Volume \nto be Pumped"() -> (w5946:dbl)
                            n5563 = local read "Volume of Syringe"() -> (w5949:dbl)
                            n5564 = call "RPickUp(SubVI).vi"("Volume to be picked up"=w5946, "Volume of Syringe"=w5949, "Resolution of PickUP"=w5947, "PickUp Flow Rate (ul/min)"=w5948, "VISA Refnum in"=w5950) -> ()  [unwired: 6 in, 1 out]
                            n5565 = local write "SEC On"(TRUE ("SEC On")) -> ()
                          }
                          frame #24 {
                            n5566 = local read "Stopper that ends \nthe main loops"() -> (w5951:bool)
                            n5567 = local read "VISA Refnum in\nfor Pump"() -> (w5952:refnum<visa-resource-name>)
                            n5568 = case shown="True" w5951 {
                              frame False {
                              }
                              frame True {
                                n5569 = local read "VISA Refnum in\nfor Pump"() -> (w5953:refnum<visa-resource-name>)
                                n5570 = call "HardStopCurrentProcess (SubVI).vi"("VISA Refnum in"=w5953) -> ()  [unwired: 11 in]
                              }
                            }
                            n5571 = call "ProcessCompletionWaiter (SubVI).vi"("VISA Refnum in"=w5952) -> ()  [unwired: 11 in]
                          }
                          frame #25 {
                            # "Reads the initial Plunger Position for computing the volume dispensed"
                            n5572 = local read "VISA Refnum in\nfor Pump"() -> (w5955:refnum<visa-resource-name>)
                            n5573 = call "AbsolutePlungerPosition (SubVI).vi"("VISA Refnum in"=w5955) -> ("Plunger Position"=w5954:i32)  [unwired: 10 in]
                            n5574 = local write "Initial Plunger Position"(w5954) -> ()
                          }
                          frame #26 {
                            # "Switch to Port-10"
                            # "Port-10 of the pump is conncted to column-2 of chip"
                            n5575 = local read "VISA Refnum in\nfor Pump"() -> (w5957:refnum<visa-resource-name>)
                            n5576 = call "PortChanger (SubVI).vi"("Port Number"="10", "VISA Refnum in"=w5957) -> ()  [unwired: 10 in]
                          }
                          frame #27 {
                            n5577 = local read "Stopper that ends \nthe main loops"() -> (w5958:bool)
                            n5578 = local read "VISA Refnum in\nfor Pump"() -> (w5959:refnum<visa-resource-name>)
                            n5579 = call "ProcessCompletionWaiter (SubVI).vi"("VISA Refnum in"=w5959) -> ()  [unwired: 11 in]
                            n5580 = case shown="True" w5958 {
                              frame False {
                              }
                              frame True {
                                n5581 = local read "VISA Refnum in\nfor Pump"() -> (w5960:refnum<visa-resource-name>)
                                n5582 = call "HardStopCurrentProcess (SubVI).vi"("VISA Refnum in"=w5960) -> ()  [unwired: 11 in]
                              }
                            }
                          }
                          frame #28 {
                            # "Keeps the AMF valve after column-1 open and valve after column-2 closed"
                            n5583 = local read "Buffer-C2 Dispense\nFlow Rate (ul/min)"() -> (w5973:dbl)
                            n5584 = local read "Buffer-C2 Pumping\nResolution"() -> (w5972:T2)
                            n5585 = local read "VISA Refnum in\nfor Pump"() -> (w5975:refnum<visa-resource-name>)
                            n5586 = local write "Pause Data Collection"(FALSE ("Pause Data Collection")) -> ()
                            n5587 = local read "Volume of Syringe"() -> (w5974:dbl)
                            n5588 = call "GoToAbsolutePosition(SubVI).vi"("Absolute Volume Position in Syringe (in ul)"=0.0 ("Volume to be Dispensed"), "Volume of Syringe"=w5974, "Resolution of Pumping"=w5972, "Flow Rate (ul/min)"=w5973, "VISA Refnum in"=w5975) -> ()  [unwired: 6 in, 1 out]
                            n5589 = local write "Valve V1 Open"(FALSE ("Valve V1 Open")) -> ()
                            n5590 = local write "Valve V2 Open"(TRUE ("Valve V2 Open")) -> ()
                            n5591 = local write "Valve V3 Open"(TRUE ("Valve V3 Open")) -> ()
                            n5592 = local write "Valve V4 Open"(FALSE ("Valve V4 Open")) -> ()
                            n5593 = local write "External Valve \nOpen"(TRUE ("External Valve \nOpen")) -> ()
                            n5594 = local write "Valve V8 Open"(FALSE ("Valve V8 Open")) -> ()
                            n5595 = local write "Valve V5 Open"(FALSE ("Valve V5 Open")) -> ()
                            n5596 = local write "Valve V6 Open"(FALSE ("Valve V6 Open")) -> ()
                            n5597 = local write "Valve V7 Open"(FALSE ("Valve V7 Open")) -> ()
                          }
                          frame #29 {
                            n5598 = local read "Initial Plunger Position"() -> (w5979:dbl)
                            n5599 = local read "Buffer-C2 Pumping\nResolution"() -> (w5978:T2)
                            n5600 = local read "VISA Refnum in\nfor Pump"() -> (w5980:refnum<visa-resource-name>)
                            n5601 = local read "Volume of Syringe"() -> (w5977:dbl)
                            n5602 = while {
                              tunnel: w5979 -> [w5986]
                              tunnel: w5980 -> [w5985]
                              tunnel: w5978 -> [w5984]
                              tunnel: w5977 -> [w5983]
                              stop <- w5981 stop-if-true
                              n5603 = Wait (ms)(milliseconds to wait=u32 100) -> ()  [unwired: 1 out]
                              n5604 = stacked-sequence {
                                tunnel: w5986 -> [w5992 _]
                                tunnel: w5985 -> [w5991 w6018]
                                tunnel: w5984 -> [w5990 _]
                                tunnel: w5983 -> [w5989 _]
                                tunnel: [_ w6014] -> w5981
                                frame #0 {
                                n5605 = call "AbsolutePlungerPosition (SubVI).vi"("VISA Refnum in"=w5991) -> ("Plunger Position"=w5988:i32)  [unwired: 10 in]
                                n5606 = case shown="\"Standard Pumping\", Default" w5990 {
                                tunnel: w5992 -> [w5997 w6006]
                                tunnel: w5988 -> [w5998 w6005]
                                tunnel: [w5996 w6003] -> w5987
                                tunnel: w5989 -> [w5995 w6004]
                                frame "Standard Pumping", Default {
                                n5607 = Subtract(x=w5997, y=w5998) -> (x-y=w5994:dbl)
                                n5608 = Absolute Value(x=w5994) -> (abs(x)=w5993:dbl)
                                n5609 = Multiply(x=w5993, y=w5995) -> (x*y=w6000:dbl)
                                n5610 = Divide(x=w6000, y=3000.0) -> (x/y=w5996:dbl)
                                }
                                frame "High Resolution Pumping" {
                                n5611 = Subtract(x=w6006, y=w6005) -> (x-y=w6002:dbl)
                                n5612 = Absolute Value(x=w6002) -> (abs(x)=w6001:dbl)
                                n5613 = Multiply(x=w6001, y=w6004) -> (x*y=w6008:dbl)
                                n5614 = Divide(x=w6008, y=24000.0) -> (x/y=w6003:dbl)
                                }
                                }
                                n5615 = local write "Volume being Injected \nin this process"(w5987) -> ()
                                }
                                frame #1 {
                                n5616 = local read "Stopper that ends \nthe main loops"() -> (w6015:bool)
                                n5617 = local read "Divert Buffer-C \ninto Column-2"() -> (w6016:bool)
                                n5618 = local read "Volume being Injected \nin this process"() -> (w6013:dbl)
                                n5619 = call "LSPOneStatus (SubVI).vi"("VISA Refnum in"=w6018) -> ("read buffer"=w6020:string)  [unwired: 10 in]
                                n5620 = call <vilib>:"Trim Whitespace.vi"("string"=w6020) -> ("trimmed string"=w6019:string)  [unwired: 1 in]
                                n5621 = Equal?(x=w6019, y="/0`\u0003") -> (x = y?=w6017:bool)
                                n5622 = Or(x=w6016, y=w6015) -> (x .or. y?=w6011:bool)
                                n5623 = Greater Or Equal?(x=w6013, y=2.0) -> (x >= y?=w6010:bool)
                                n5624 = Or(x=w6011, y=w6010) -> (x .or. y?=w6009:bool)
                                n5625 = Or(x=w6017, y=w6009) -> (x .or. y?=w6014:bool)
                                }
                              }
                            }
                            n5626 = local read "Stopper that ends \nthe main loops"() -> (w5976:bool)
                            n5627 = case shown="True" w5976 {
                              frame False {
                              }
                              frame True {
                                n5628 = local read "VISA Refnum in\nfor Pump"() -> (w6022:refnum<visa-resource-name>)
                                n5629 = call "HardStopCurrentProcess (SubVI).vi"("VISA Refnum in"=w6022) -> ()  [unwired: 11 in]
                              }
                            }
                          }
                          frame #30 {
                            # "Keeps the on-chip valves V4, V5 and V7 open"
                            # "Keeps the AMF valve after column-1 closed and valve after column-2 open"
                            n5630 = local write "Divert Buffer-C \ninto Column-2"(FALSE ("Divert Buffer-C \ninto Column-2")) -> ()
                            n5631 = local write "Valve V3 Open"(TRUE ("Valve V3 Open")) -> ()
                            n5632 = local write "Valve V2 Open"(FALSE ("Valve V2 Open")) -> ()
                            n5633 = local write "Valve V1 Open"(FALSE ("Valve V1 Open")) -> ()
                            n5634 = local write "Valve V4 Open"(TRUE ("Valve V4 Open")) -> ()
                            n5635 = local write "External Valve \nOpen"(FALSE ("External Valve \nOpen")) -> ()
                            n5636 = local write "Valve V5 Open"(TRUE ("Valve V5 Open")) -> ()
                            n5637 = local write "Valve V6 Open"(FALSE ("Valve V6 Open")) -> ()
                            n5638 = local write "Valve V8 Open"(FALSE ("Valve V8 Open")) -> ()
                            n5639 = local write "Valve V7 Open"(TRUE ("Valve V7 Open")) -> ()
                          }
                          frame #31 {
                            n5640 = local read "Initial Plunger Position"() -> (w6036:dbl)
                            n5641 = local read "Buffer-C2 Pumping\nResolution"() -> (w6035:T2)
                            n5642 = local read "VISA Refnum in\nfor Pump"() -> (w6037:refnum<visa-resource-name>)
                            n5643 = local read "Volume of Syringe"() -> (w6034:dbl)
                            n5644 = while {
                              tunnel: w6036 -> [w6043]
                              tunnel: w6037 -> [w6042]
                              tunnel: w6035 -> [w6041]
                              tunnel: w6034 -> [w6040]
                              stop <- w6038 stop-if-true
                              n5645 = Wait (ms)(milliseconds to wait=u32 100) -> ()  [unwired: 1 out]
                              n5646 = stacked-sequence {
                                tunnel: w6043 -> [w6049 _]
                                tunnel: w6042 -> [w6048 w6071]
                                tunnel: w6041 -> [w6047 _]
                                tunnel: w6040 -> [w6046 _]
                                tunnel: [_ w6069] -> w6038
                                frame #0 {
                                n5647 = call "AbsolutePlungerPosition (SubVI).vi"("VISA Refnum in"=w6048) -> ("Plunger Position"=w6045:i32)  [unwired: 10 in]
                                n5648 = case shown="\"Standard Pumping\", Default" w6047 {
                                tunnel: w6049 -> [w6054 w6063]
                                tunnel: w6045 -> [w6055 w6062]
                                tunnel: [w6053 w6060] -> w6044
                                tunnel: w6046 -> [w6052 w6061]
                                frame "Standard Pumping", Default {
                                n5649 = Subtract(x=w6054, y=w6055) -> (x-y=w6051:dbl)
                                n5650 = Absolute Value(x=w6051) -> (abs(x)=w6050:dbl)
                                n5651 = Multiply(x=w6050, y=w6052) -> (x*y=w6057:dbl)
                                n5652 = Divide(x=w6057, y=3000.0) -> (x/y=w6053:dbl)
                                }
                                frame "High Resolution Pumping" {
                                n5653 = Subtract(x=w6063, y=w6062) -> (x-y=w6059:dbl)
                                n5654 = Absolute Value(x=w6059) -> (abs(x)=w6058:dbl)
                                n5655 = Multiply(x=w6058, y=w6061) -> (x*y=w6065:dbl)
                                n5656 = Divide(x=w6065, y=24000.0) -> (x/y=w6060:dbl)
                                }
                                }
                                n5657 = local write "Volume being Injected \nin this process"(w6044) -> ()
                                }
                                frame #1 {
                                n5658 = call "LSPOneStatus (SubVI).vi"("VISA Refnum in"=w6071) -> ("read buffer"=w6073:string)  [unwired: 10 in]
                                n5659 = call <vilib>:"Trim Whitespace.vi"("string"=w6073) -> ("trimmed string"=w6072:string)  [unwired: 1 in]
                                n5660 = Equal?(x=w6072, y="/0`\u0003") -> (x = y?=w6070:bool)
                                n5661 = local read "Stopper that ends \nthe main loops"() -> (w6067:bool)
                                n5662 = local read "Divert Sample \nonto Grid"() -> (w6068:bool)
                                n5663 = Or(x=w6068, y=w6067) -> (x .or. y?=w6066:bool)
                                n5664 = Or(x=w6070, y=w6066) -> (x .or. y?=w6069:bool)
                                }
                              }
                            }
                            n5665 = local read "Stopper that ends \nthe main loops"() -> (w6033:bool)
                            n5666 = case shown="True" w6033 {
                              frame False {
                              }
                              frame True {
                                n5667 = local read "VISA Refnum in\nfor Pump"() -> (w6075:refnum<visa-resource-name>)
                                n5668 = call "HardStopCurrentProcess (SubVI).vi"("VISA Refnum in"=w6075) -> ()  [unwired: 11 in]
                              }
                            }
                          }
                          frame #32 {
                            n5669 = local read "Volume being Injected \nin this process"() -> (w6078:dbl)
                            n5670 = local read "VISA Refnum in\nfor Pump"() -> (w6080:refnum<visa-resource-name>)
                            n5671 = call "AbsolutePlungerPosition (SubVI).vi"("VISA Refnum in"=w6080) -> ("Plunger Position"=w6079:i32)  [unwired: 10 in]
                            n5672 = local write "Pause Data Collection"(TRUE) -> ()
                            n5673 = local write "True Volume being \ninjected in this\nprocess"(w6078) -> ()
                            n5674 = local write "Position\nNow"(w6079) -> ()
                            n5675 = Wait (ms)(milliseconds to wait=u32 500) -> ()  [unwired: 1 out]
                          }
                          frame #33 {
                            # "Sample Deposition onto EM-Grid"
                            n5676 = local read "Divert Sample \nonto Grid"() -> (w6081:bool)
                            n5677 = case shown="True" w6081 {
                              frame False {
                              }
                              frame True {
                                n5678 = stacked-sequence {
                                frame #0 {
                                # "Discard the initial volume of fluid that is present in the channel prior to detection"
                                n5679 = local read "Buffer-C2 Pumping\nResolution"() -> (w6094:T2)
                                n5680 = local read "Initial Plunger Position"() -> (w6093:dbl)
                                n5681 = local read "VISA Refnum in\nfor Pump"() -> (w6095:refnum<visa-resource-name>)
                                n5682 = local read "Position\nNow"() -> (w6091:dbl)
                                n5683 = local read "Volume of Syringe"() -> (w6092:dbl)
                                n5684 = local write "Pause Data Collection"(FALSE) -> ()
                                n5685 = while {
                                tunnel: w6095 -> [w6105]
                                tunnel: w6094 -> [w6104]
                                tunnel: w6093 -> [w6100]
                                tunnel: w6092 -> [w6103]
                                tunnel: w6091 -> [w6099]
                                stop <- w6101 stop-if-true
                                n5686 = stacked-sequence {
                                tunnel: w6105 -> [w6111 w6133 w6165]
                                tunnel: w6104 -> [w6110 w6132 _]
                                tunnel: w6100 -> [w6108 _ _]
                                tunnel: w6103 -> [w6107 w6130 _]
                                tunnel: [_ _ w6159] -> w6101
                                tunnel: w6099 -> [_ w6128 _]
                                frame #0 {
                                # "From here on 'True Volume being injected \nin this process' represents the true total \nvolume in this process"
                                n5687 = call "AbsolutePlungerPosition (SubVI).vi"("VISA Refnum in"=w6111) -> ("Plunger Position"=w6109:i32)  [unwired: 10 in]
                                n5688 = case shown="..\"Standard Pumping\"" w6110 {
                                tunnel: w6109 -> [w6119 w6127]
                                tunnel: w6108 -> [w6118 w6126]
                                tunnel: w6107 -> [w6115 w6123]
                                tunnel: [w6112 w6120] -> w6106
                                frame .."Standard Pumping" {
